vi "Substitution.vi"(10 "actual theta":dbl, 11 "cluster":cluster{"velocity":dbl, "target theta":dbl}) -> (3 "output cluster":cluster{"velocity":dbl, "travel angle":dbl})   [LabVIEW 2020]
uses:
  <vilib>/Analysis/coordinate.llb/Angle Range (Degree).ctl
  <vilib>/Analysis/coordinate.llb/Angle Units.ctl
  <vilib>/Analysis/coordinate.llb/Wrap Angle (scalar).vi
  <vilib>/Analysis/NI_AAL_Angle.lvlib
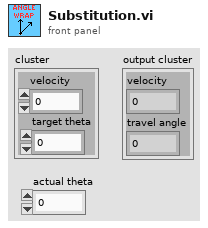
[diagram p1: front panel]
types:
  T1 = typedef "NI_AAL_Angle.lvlib/Angle Units.ctl" = i32
  T2 = typedef "NI_AAL_Angle.lvlib/Angle Range (Degree).ctl" = u16
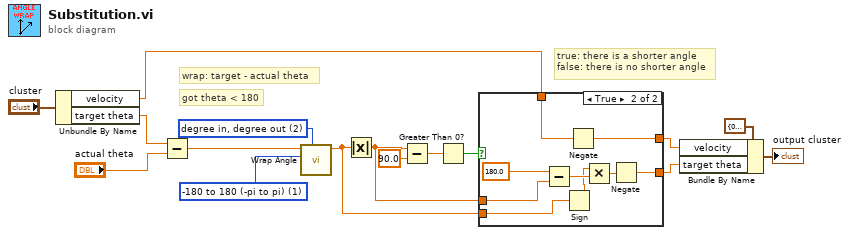
[diagram p0: block diagram]
diagram:
  w15 = T1 2 items=["radian in, radian out", "radian in, degree out", "degree in, degree out", "degree in, radian out"] ("angle units")
  w16 = T2 1 items=["none", "-180 to 180 (-pi to pi)", "0 to 360 (0 to 2pi)"] ("angle range")
  # "true: there is a shorter angle\nfalse: there is no shorter angle"
  # "got theta < 180"
  # "wrap: target - actual theta"
  n1 = Unbundle By Name("cluster") -> ("velocity"=w8:dbl, "target theta"=w13:dbl)
  n2 = Subtract(x=w13, y="actual theta") -> (x-y=w11:dbl)
  n3 = call-poly <vilib>:"Wrap Angle.vi"("angle units"=w15, "angle range"=w16, "angle in"=w11) -> ("angle out"=w1:dbl)  [unwired: 7 in, 1 out]
  n4 = Absolute Value(x=w1) -> (abs(x)=w2:dbl)
  n5 = Subtract(x=w2, y=90.0) -> (x-y=w7:dbl)
  n6 = Greater Than 0?(x=w7) -> (x > 0?=w9:bool)
  n7 = case shown="True" w9 {
    tunnel: w8 -> [w18 w27]
    tunnel: [w18 w26] -> w6
    tunnel: w2 -> [w17 w23]
    tunnel: [w17 w25] -> w3
    tunnel: w1 -> [_ w20]
    frame False {
    }
    frame True {
      n8 = Subtract(x=180.0, y=w23) -> (x-y=w21:dbl)
      n9 = Sign(1:w20) -> (0:w19:dbl)
      n10 = Negate(x=w27) -> (-x=w26:dbl)
      n11 = Multiply(x=w19, y=w21) -> (x*y=w22:dbl)
      n12 = Negate(x=w22) -> (-x=w25:dbl)
    }
  }
  n13 = Bundle By Name(cluster=cluster{"velocity":dbl, "target theta":dbl} {"velocity"=0.0, "target theta"=0.0}, "velocity"=w6, "target theta"=w3) -> (→"output cluster":cluster{"velocity":dbl, "target theta":dbl})
